vi "FRP.vi"(0 "System no.":i32=1 min=1 max=4 step=1, 2 "Routinename":string[](array[string]), 3 "Option":i32[](array[numeric]), 5 "error in":errorcluster) -> (19 "error out":errorcluster)   [LabVIEW 2020]
doc: "Stops, pauses or resumes the given fast alignment routine(s).\n\nC-887, E-727.AS: Option can be\n0 - stop given routine\n\nE-712: Option can be\n0 - stop given routine\n1 - pause given routine\n2 - resume given routine\n\nC-887, E-712, E-727.AS:"
panel:
  # "Stops, pauses or resumes the given fast alignment procedure(s)."
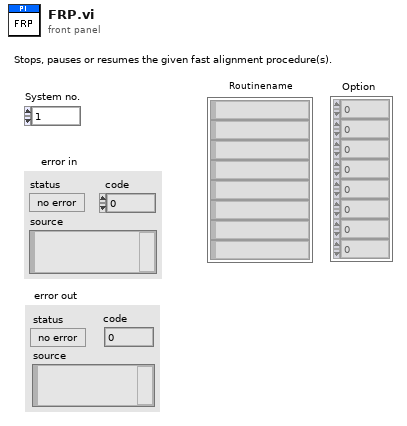
[diagram p1: front panel]
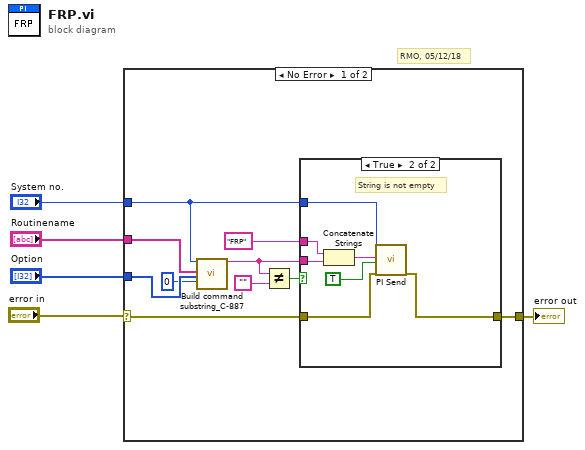
[diagram p0: block diagram]
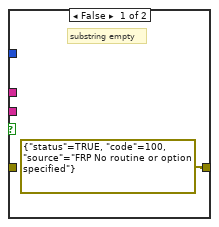
[diagram p2: hidden frame]
diagram:
  # "RMO, 05/12/18"
  n1 = case shown="No Error" "error in" {
    selector: "error in" -> [w6 w24]
    tunnel: [w15 w24] -> w5
    tunnel: "Option" -> [w12 _]
    tunnel: "System no." -> [w10 _]
    tunnel: "Routinename" -> [w11 _]
    frame No Error {
      n2 = call "Build command substring_C-887.vi"("System no."=w10, "Affected axes"=w11, "Parameters"=w12, "No. of digits"=i16 0) -> ("Command substring"=w13:string)  [unwired: 3 in, 12 out]
      n3 = Not Equal?(x=w13, y="") -> (x != y?=w7:bool)
      n4 = case shown="True" w7 {
        tunnel: w13 -> [_ w23]
        tunnel: [errorcluster {"status"=TRUE, "code"=100, "source"="FRP No routine or option specified"} ("error out") w17] -> w15
        tunnel: w6 -> [_ w20]
        tunnel: w10 -> [_ w19]
        tunnel: "FRP" -> [_ w18]
        frame False {
          # "substring empty"
        }
        frame True {
          # "String is not empty"
          n5 = Concatenate Strings(w18, w23) -> (w21:string)
          n6 = call "PI Send.vi"("System no."=w19, "String to send"=w21, "Attach termination char.?"=TRUE ("Attach Linefeed?"), "error in"=w20) -> ("error out"=w17:errorcluster)  [unwired: 2 in, 13 out]
        }
      }
    }
    frame Error {
    }
  }
  "error out" <- w5
